vi "子VI-读取缺陷测量长宽和面积.vi"(10 "Particle Reports (Pixels)":T1(array[cluster]) {"Orientation" format="%.2f"; "Dimensions"."Height" format="%.2f"; "Dimensions"."Width" format="%.2f"; "Center of Mass"."Y" format="%.2f"; "Center of Mass"."X" format="%.2f"; "Bounding Rect"."Bottom" format="%.2f"; "Bounding Rect"."Right" format="%.2f"; "Bounding Rect"."Top" format="%.2f"; "Bounding Rect"."Left" format="%.2f"; "Number of Holes" format="%.2f"; "Area" format="%.2f"}) -> (2 "测量结果":dbl[][](array[numeric]))   [LabVIEW 2018]
panel:
  out "补五列空数字":dbl[](array[numeric])
  out "高":dbl[](array[numeric])
  out "宽":dbl[](array[numeric])
  out "面积":dbl[](array[numeric])
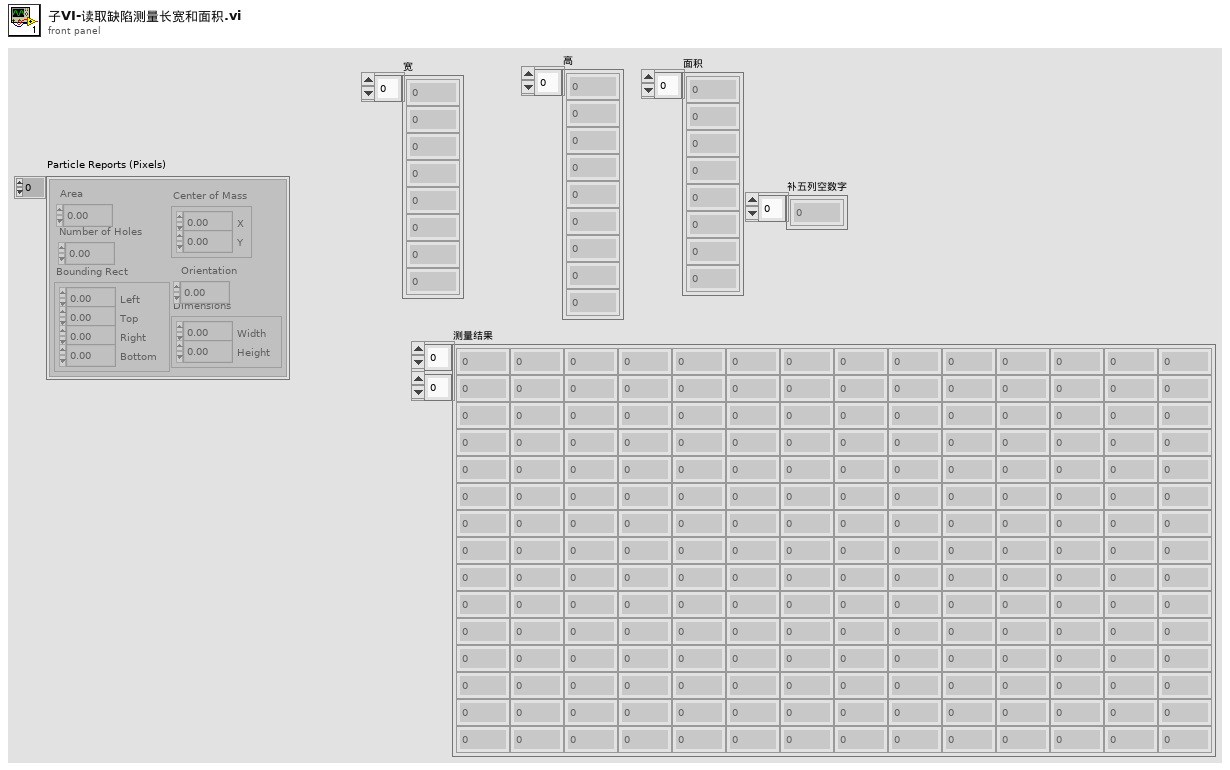
[diagram p1: front panel]
types:
  T1 = cluster{"Area":dbl, "Number of Holes":dbl, "Bounding Rect":cluster{"Left":dbl, "Top":dbl, "Right":dbl, "Bottom":dbl}, "Center of Mass":cluster{"X":dbl, "Y":dbl}, "Orientation":dbl, "Dimensions":cluster{"Width":dbl, "Height":dbl}}[]
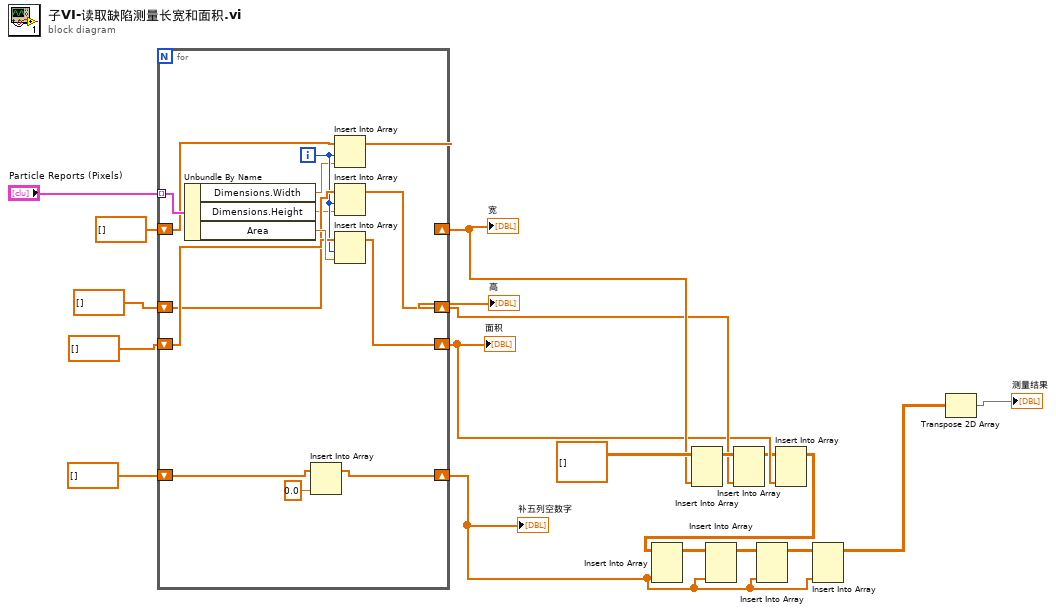
[diagram p0: block diagram]
diagram:
  n1 = for {
    tunnel: "Particle Reports (Pixels)" -> [w32] mode=indexing
    shift-right: [w29] -> w10
    shift-left: dbl[] [] ("数组") -> [w30]
    shift-right: [w24] -> w13
    shift-left: dbl[] [] ("数组") -> [w26]
    shift-right: [w25] -> w11
    shift-left: dbl[] [] ("数组") -> [w28]
    shift-right: [w19] -> w2
    shift-left: dbl[] [] ("数组") -> [w21]
    i -> [w27]
    n2 = Unbundle By Name(w32) -> ("Dimensions.Width"=w22:dbl, "Dimensions.Height"=w23:dbl, "Area"=w31:dbl)
    n3 = Insert Into Array(array=w21, new element=0.0 ("新元素/子数组")) -> (w19:dbl[])  [unwired: 1 in]
    n4 = Insert Into Array(array=w26, index=w27, new element=w22) -> (w24:dbl[])
    n5 = Insert Into Array(array=w28, index=w27, new element=w23) -> (w25:dbl[])
    n6 = Insert Into Array(array=w30, index=w27, new element=w31) -> (w29:dbl[])
  }
  "面积" <- w10
  "宽" <- w13
  "高" <- w11
  "补五列空数字" <- w2
  n7 = Insert Into Array(array=dbl[][] [] ("数组"), new element=w13) -> (w12:dbl[][])  [unwired: 2 in]
  n8 = Insert Into Array(array=w12, new element=w11) -> (w9:dbl[][])  [unwired: 2 in]
  n9 = Insert Into Array(array=w9, new element=w10) -> (w6:dbl[][])  [unwired: 2 in]
  n10 = Insert Into Array(array=w6, new element=w2) -> (w5:dbl[][])  [unwired: 2 in]
  n11 = Insert Into Array(array=w5, new element=w2) -> (w4:dbl[][])  [unwired: 2 in]
  n12 = Insert Into Array(array=w4, new element=w2) -> (w3:dbl[][])  [unwired: 2 in]
  n13 = Insert Into Array(array=w3, new element=w2) -> (w1:dbl[][])  [unwired: 2 in]
  n14 = Transpose 2D Array(2D array=w1) -> (transposed array=→"测量结果":dbl[][])
